vi "Read DataMap.vi"(8 "error in (no error)":errorcluster, 11 "gController in":refnum<class "gController.lvclass">) -> (0 "error out":errorcluster, 2 "DataMap":refnum<data-value>, 3 "gController out":refnum<class "gController.lvclass">)   [LabVIEW 2016, in "Controller.lvlib" / "gController.lvclass"]
uses:
  gController.lvclass
  gController.lvclass/gController.ctl
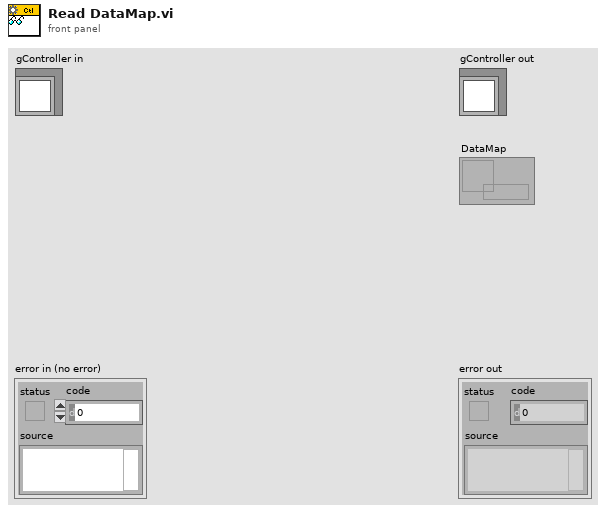
[diagram p1: front panel]
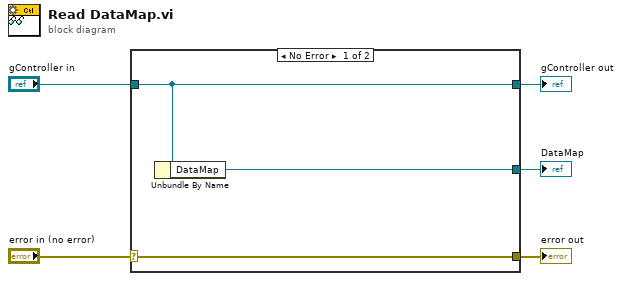
[diagram p0: block diagram]
diagram:
  n1 = case shown="No Error" "error in (no error)" {
    selector: "error in (no error)" -> [w8 w9]
    tunnel: [w8 w9] -> w4
    tunnel: [w7 w10] -> w2
    tunnel: "gController in" -> [w7 w10]
    tunnel: [w6 _] -> w1
    frame No Error {
      n2 = Unbundle By Name(w7) -> ("DataMap"=w6:refnum<data-value>)
    }
    frame Error {
    }
  }
  "error out" <- w4
  "gController out" <- w2
  "DataMap" <- w1
